vi "Remove.vi"(8 "error in (no error)":errorcluster, 10 "Test to Remove":string, 11 "LUnit Test Suite In":refnum<class "LUnit Test Suite.lvclass">) -> (0 "error out":errorcluster, 3 "LUnit Test Suite Out":refnum<class "LUnit Test Suite.lvclass">)   [LabVIEW 2020, in "LUnit Test Suite.lvclass"]
uses:
  LUnit Test Suite.lvclass
  C:/git/astemes-lunit/source/Core/Runnable/Runnable.lvclass
  LUnit Test Suite.lvclass/LUnit Test Suite.ctl
  Core/Runnable/Runnable.lvclass
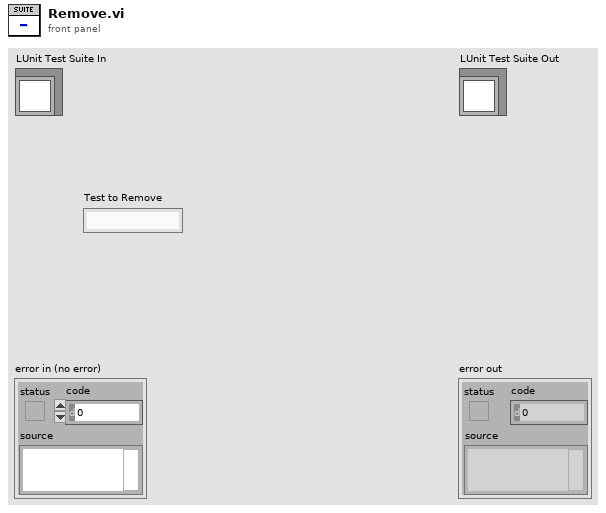
[diagram p1: front panel]
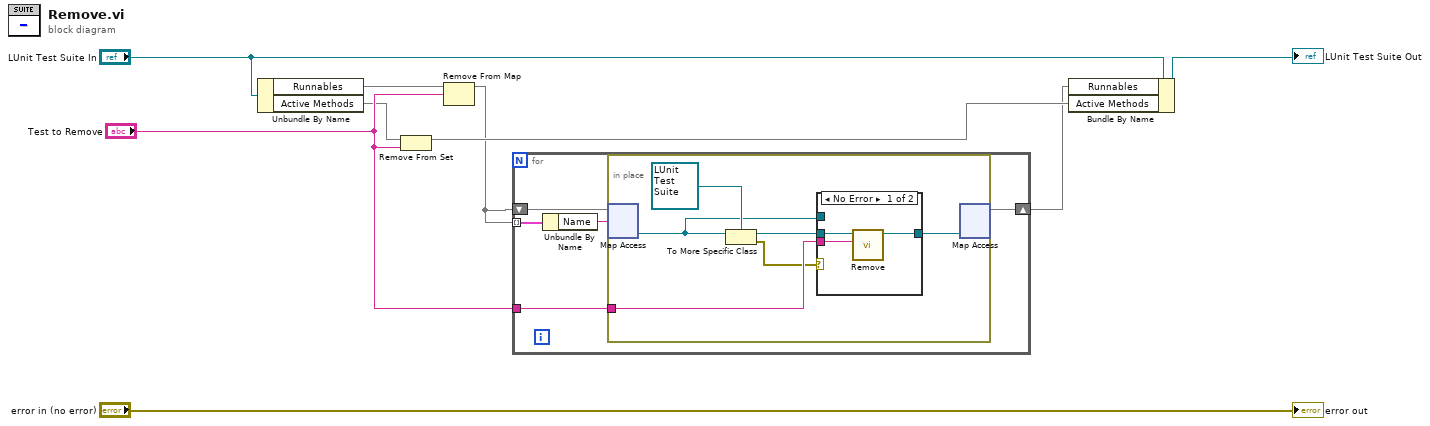
[diagram p0: block diagram]
diagram:
  n1 = Unbundle By Name("LUnit Test Suite In") -> ("Runnables"=w5:map{string, refnum<class "Runnable.lvclass">}, "Active Methods"=w4:set{string})
  n2 = Remove From Set(10:"Test to Remove", 11:w4) -> (3:w3:set{string})  [unwired: 1 out]
  n3 = Remove From Map(10:"Test to Remove", 11:w5) -> (3:w2:map{string, refnum<class "Runnable.lvclass">})  [unwired: 2 out]
  n4 = for {
    tunnel: w2 -> [w13] mode=indexing
    shift-right: [w10] -> w1
    shift-left: w2 -> [w14]
    tunnel: "Test to Remove" -> [w11]
    n5 = Unbundle By Name(w13) -> ("Name"=w12:string)
    n6 = in-place {
      in-place-border: w11 -> [w19]
      n7 = in-place-map #1(w14, w12) -> (w15:refnum<class "Runnable.lvclass">)  [unwired: 1 in, 1 out]
      n8 = To More Specific Class(target class=refnum<class "LUnit Test Suite.lvclass"> refnum ("LUnit Test Suite.lvclass"), reference=w15) -> (specific class reference=w16:refnum<class "LUnit Test Suite.lvclass">, error out=w17:errorcluster)  [unwired: 1 in]
      n9 = case shown="No Error" w17 {
        tunnel: w16 -> [w23 _]
        tunnel: w19 -> [w22 _]
        tunnel: [w21 w24] -> w18
        tunnel: w15 -> [_ w24]
        frame No Error {
          n10 = call "Remove.vi"("Test to Remove"=w22, "LUnit Test Suite In"=w23) -> ("LUnit Test Suite Out"=w21:refnum<class "LUnit Test Suite.lvclass">)  [unwired: 8 in, 1 out]
        }
        frame Error {
        }
      }
      n11 = in-place-map #1(w18) -> (w10:map{string, refnum<class "Runnable.lvclass">})  [unwired: 1 in, 2 out]
    }
  }
  n12 = Bundle By Name(cluster="LUnit Test Suite In", "Runnables"=w1, "Active Methods"=w3) -> (→"LUnit Test Suite Out":refnum<class "LUnit Test Suite.lvclass">)
  "error out" <- "error in (no error)"
